vi "Write.vi"(4 "Error In":errorcluster, 6 "Plugin Name":T1, 7 "Sample Period (msec)":i32) -> (0 "Error Out":errorcluster, 2 "Plugin Name Out":T1, 3 "Sample Period Out (msec)":i32)   [LabVIEW 2020, in "Sample Rate.lvlib"]
uses:
  Sample Rate.lvlib
  toolbox/Debugging/Debugging.lvlib
  _libraries/Startup Processes/_typedefs/Subpanel Names.ctl
  _libraries/Startup Processes/Startup Processes.lvlib
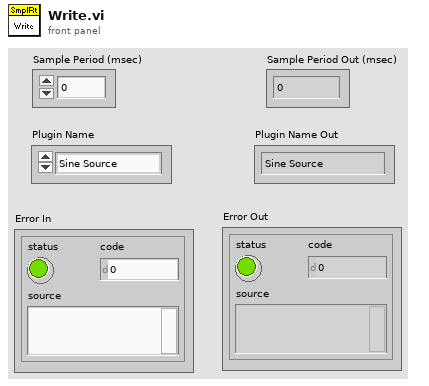
[diagram p1: front panel]
types:
  T1 = typedef "Startup Processes.lvlib/Subpanel Names.ctl" = enum16{"Sine Source", "Ramp Source", "Hen House TC", "Dog House TC", "Out House TC"}
  T2 = typedef "Sample Rate.lvlib/data.ctl" = cluster{"Sine Sample Period":i32, "Ramp Sample Period":i32}
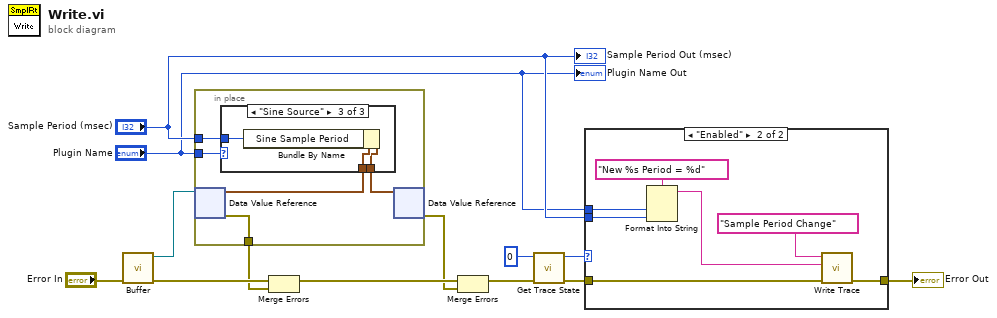
[diagram p0: block diagram]
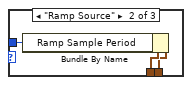
[diagram p4: hidden frame]
diagram:
  n1 = call "Buffer.vi"("Error In"="Error In") -> ("Error Out"=w11:errorcluster, "DVR"=w13:refnum<data-value>)  [unwired: 5 in]
  n2 = in-place {
    in-place-border: "Sample Period (msec)" -> [w15]
    in-place-border: [w18] -> w2
    in-place-border: "Plugin Name" -> [w14]
    n3 = in-place-dvr #1(w13) -> (w17:T2, w18:errorcluster)
    n4 = case shown="\"Sine Source\"" w14 {
      tunnel: w17 -> [w19 w22 w25]
      tunnel: [w19 w21 w24] -> w16
      tunnel: w15 -> [_ w20 w23]
      frame Default {
      }
      frame "Ramp Source" {
        n5 = Bundle By Name(cluster=w22, "Ramp Sample Period"=w20) -> (w21:T2)
      }
      frame "Sine Source" {
        n6 = Bundle By Name(cluster=w25, "Sine Sample Period"=w23) -> (w24:T2)
      }
    }
    n7 = in-place-dvr #1(w16) -> (w1:errorcluster)  [unwired: 1 out]
  }
  n8 = Merge Errors(w11, w2) -> (w10:errorcluster)
  n9 = Merge Errors(w10, w1) -> (w6:errorcluster)
  n10 = call "Get Trace State.vi"("Error In"=w6, "Trace Point Index"=0) -> ("Error Out"=w7:errorcluster, "Trace Point State"=w8:enum16{"Disabled", "Enabled"})  [unwired: 4 in]
  n11 = case shown="\"Enabled\"" w8 {
    tunnel: w7 -> [w26 w33]
    tunnel: [w26 w32] -> w4
    tunnel: "Sample Period (msec)" -> [_ w30]
    tunnel: "Plugin Name" -> [_ w27]
    frame "Disabled" {
    }
    frame "Enabled" {
      n12 = Format Into String(format string="New %s Period = %d", w27, w30) -> (resulting string=w29:string)  [unwired: 2 in, 1 out]
      n13 = call "Write Trace.vi"("Error In"=w33, "Trace Data"=w29, "Trace Point Name"="Sample Period Change") -> ("Error Out"=w32:errorcluster)  [unwired: 4 in]
    }
  }
  "Error Out" <- w4
  "Sample Period Out (msec)" <- "Sample Period (msec)"
  "Plugin Name Out" <- "Plugin Name"
